vi "Reset.vi"(0 "VISA resource name":refnum<visa-resource-name>, 7 "Reset Defaults (F:Dont Reset)":bool, 11 "error in (no error)":errorcluster) -> (4 "VISA resource name out":refnum<visa-resource-name>, 15 "error out":errorcluster)   [LabVIEW 2019, in "Lake Shore Cryotronics 340.lvlib"]
doc: "This VI resets the instrument, and then sends a set of default setup commands to the instrument. \n\nNOTE: If you do not want the instrument reset to its default setup state you MUST set the Reset Defaults control to FALSE."
uses:
  Lake Shore Cryotronics 340.lvlib
panel:
  # "Reset to Default State\nDon't Reset to Default State"
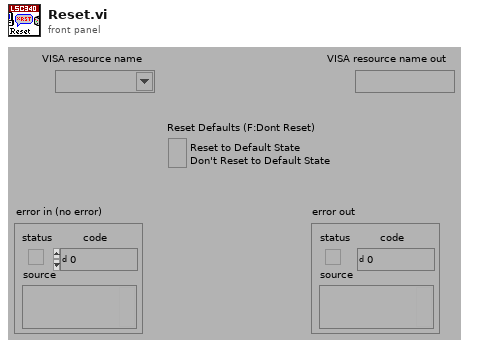
[diagram p1: front panel]
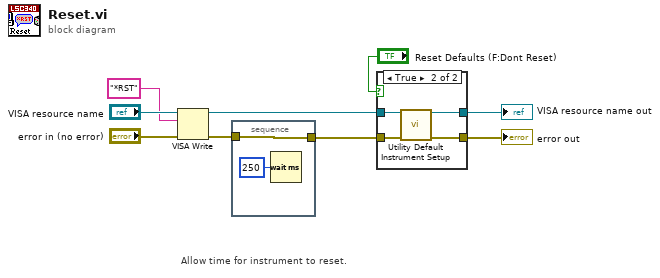
[diagram p0: block diagram]
diagram:
  # "Allow time for instrument to reset."
  n1 = VISA Write(VISA resource name="VISA resource name", write buffer="*RST" ("Reset Command"), error in (no error)="error in (no error)") -> (VISA resource name out=w2:refnum<visa-resource-name>, error out=w4:errorcluster)  [unwired: 1 out]
  n2 = stacked-sequence {
    tunnel: w4 -> [w10]
    tunnel: [w10] -> w3
    frame #0 {
      n3 = Wait (ms)(milliseconds to wait=u32 250) -> ()  [unwired: 1 out]
    }
  }
  n4 = case shown="True" "Reset Defaults (F:Dont Reset)" {
    tunnel: [w12 w17] -> w7
    tunnel: [w13 w16] -> w6
    tunnel: w3 -> [w12 w15]
    tunnel: w2 -> [w13 w14]
    frame False {
    }
    frame True {
      n5 = call "Utility Default Instrument Setup.vi"("VISA resource name"=w14, "error in (no error)"=w15) -> ("VISA resource name out"=w16:refnum<visa-resource-name>, "error out"=w17:errorcluster)  [unwired: 12 in]
    }
  }
  "error out" <- w7
  "VISA resource name out" <- w6
